vi "Delete_Device.vi"(7 "LabVIEW Web Service Request":refnum<class "Web Request.lvclass">) -> ()   [LabVIEW 2016]
uses:
  <vilib>/wsapi/Web Request.lvclass
  Device Info.ctl
  Inventory FGV Command.ctl
  <vilib>/NI_Real-Time Target Support.lvlib
panel:
  # "Use the Web Service Request input terminal to call the VIs on the Web Services palette. Do not remove it from the connector pane unless you don't need access to the palette."
  # "Each additional control wired to the connector pane will be available as an input in the URL. To include an indicator in terminal-mode output (the default setting), it must also be wired to the connector pane."
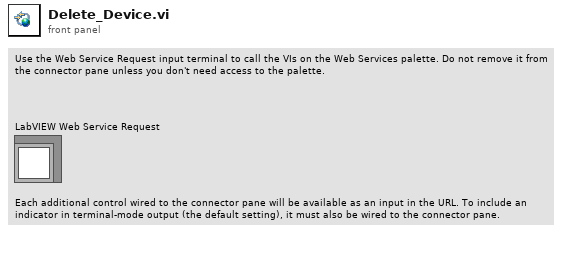
[diagram p1: front panel]
types:
  T1 = typedef "Inventory FGV Command.ctl" = enum16{"Load Items", "Check Status", "Return Items", "Check Out Items", "Add New Item", "Get All Items", "Remove Item", "Search"}
  T2 = typedef "Device Info.ctl" = cluster{"Model Number":string, "Identifier":string, "Available?":bool, "Owner":string, "Owner Email":string, "Last Activity Date":string, "Loan Purpose":string, "Department":string, "Notes":string, "Serial Number":string}
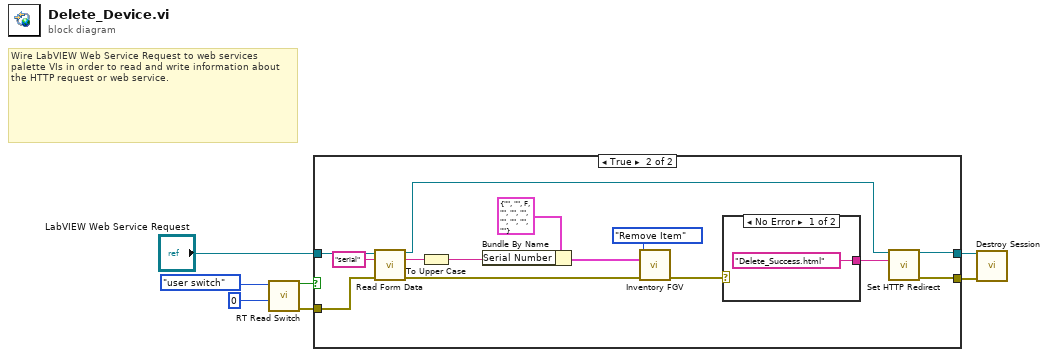
[diagram p0: block diagram]
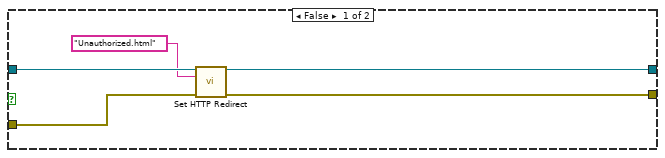
[diagram p2: hidden frame]
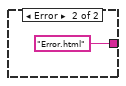
[diagram p3: hidden frame]
diagram:
  # "Wire LabVIEW Web Service Request to web services palette VIs in order to read and write information about the HTTP request or web service."
  n1 = call <vilib>:"RT Read Switch.vi"("switch ID"=0, "switch type (system switch)"=enum16{"system switch", "user switch"}."user switch") -> ("error out"=w3:errorcluster, "switch state (on/off)"=w4:bool)  [unwired: 8 in]
  n2 = case shown="True" w4 {
    tunnel: "LabVIEW Web Service Request" -> [w12 w26]
    tunnel: w3 -> [w11 w18]
    tunnel: [w9 w15] -> w1
    tunnel: [w8 w13] -> w2
    frame False {
      n3 = call <vilib>:"Set HTTP Redirect.vi"("LabVIEW Web Service Request"=w12, "redirect URL"="Unauthorized.html", "error in (no error)"=w11) -> ("LabVIEW Web Service Request out"=w8:refnum<class "Web Request.lvclass">, "error out"=w9:errorcluster)  [unwired: 11 in]
    }
    frame True {
      n4 = call <vilib>:"Read Form Data.vi"("LabVIEW Web Service Request"=w26, "key"="serial", "error in (no error)"=w18) -> ("LabVIEW Web Service Request out"=w16:refnum<class "Web Request.lvclass">, "value"=w24:string, "error out"=w19:errorcluster)  [unwired: 9 in, 1 out]
      n5 = To Upper Case(1:w24) -> (0:w22:string)
      n6 = Bundle By Name(cluster=T2 {"Model Number"="", "Identifier"="", "Available?"=FALSE, "Owner"="", "Owner Email"="", "Last Activity Date"="", "Loan Purpose"="", "Department"="", "Notes"="", "Serial Number"=""} ("Device"), "Serial Number"=w22) -> (w21:T2)
      n7 = call "Inventory FGV.vi"("error in"=w19, "Device Info"=w21, "Command"=Inventory_FGV_Command."Remove Item") -> ("error out"=w17:errorcluster)  [unwired: 5 in, 2 out]
      n8 = case shown="No Error" w17 {
        tunnel: ["Delete_Success.html" "Error.html"] -> w14
        frame No Error {
        }
        frame Error {
        }
      }
      n9 = call <vilib>:"Set HTTP Redirect.vi"("LabVIEW Web Service Request"=w16, "redirect URL"=w14) -> ("LabVIEW Web Service Request out"=w13:refnum<class "Web Request.lvclass">, "error out"=w15:errorcluster)  [unwired: 12 in]
    }
  }
  n10 = call <vilib>:"Destroy Session.vi"("LabVIEW Web Service Request"=w2, "error in (no error)"=w1) -> ()  [unwired: 12 in, 2 out]
